vi "JSON to LVObject.vi"(7 "Demo LVClass Serializer in":refnum<class "Demo LVClass Serializer.lvclass">, 8 "error in (no error)":errorcluster, 9 "Object Type":refnum<class>, 10 "Offset":i32, 11 "JSON":string) -> (0 "error out":errorcluster, 1 "Object":refnum<class>)   [LabVIEW 2019, in "Demo LVClass Serializer.lvclass"]
doc: "Convert JSON to an Object of a LabVIEW Class.\n\nThis demonstration uses an XML representation in a JSON String."
uses:
  Demo LVClass Serializer.lvclass
  vi.lib/JDP Science/JSONtext/LVClass Serializer/JSONtext LVClass Serializer.lvclass
  vi.lib/JDP Science/JSONtext/JSONtext.lvlib
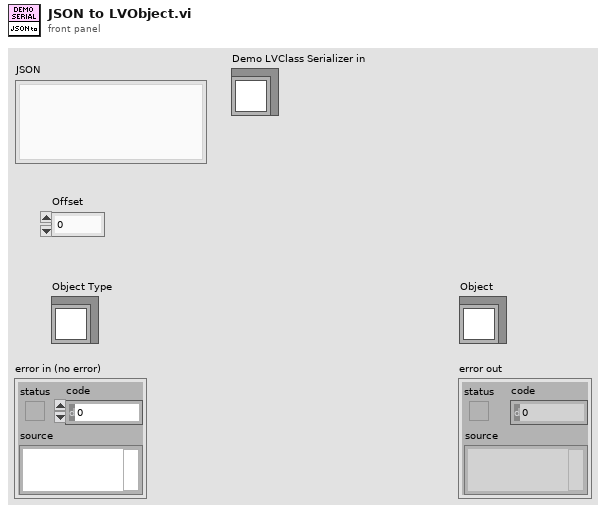
[diagram p1: front panel]
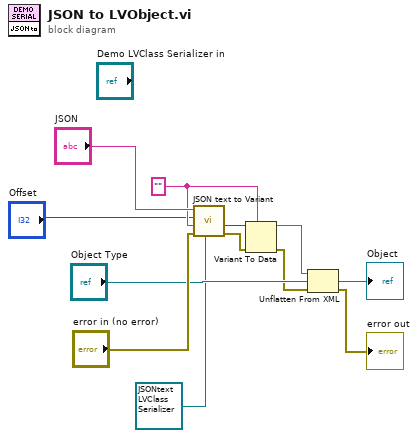
[diagram p0: block diagram]
diagram:
  w10 = ""
  n1 = call "JSON text to Variant.vi"("LVClass Serializer"=refnum<class "JSONtext LVClass Serializer.lvclass"> refnum, "error in (no error)"="error in (no error)", "Data Type"=w10, "Offset"="Offset", "JSON"="JSON") -> ("error out"=w9:errorcluster, "Variant out"=w11:variant)  [unwired: 5 in]
  n2 = Variant To Data(error in=w9, type=w10, Variant=w11) -> (data=w7:string, error out=w4:errorcluster)
  n3 = Unflatten From XML(xml string=w7, type="Object Type", error in (no error)=w4) -> (value=→"Object":refnum<class>, error out=→"error out":errorcluster)
